vi "Construct Command - Erase.vi"(8 "error in (no error)":errorcluster, 10 "Erase Configuration":T1={"Start Address"="", "End Address"="", "Reset"=TRUE}) -> (0 "error out":errorcluster, 2 "Command":string)   [LabVIEW 2016, in "JLink Commander.lvlib"]
doc: "Construct an Erase command which erases all flash sectors or a certain flash range of the current device. A device has to be specified previously. When specified, all flash between the <SAddr> and <EAddr> will be erased. By default, the device is being reset before starting the erase operation. This may be skipped by adding \"noreset\"."
uses:
  JLink Commander.lvlib
  Type Definitions/Erase Configuration.ctl
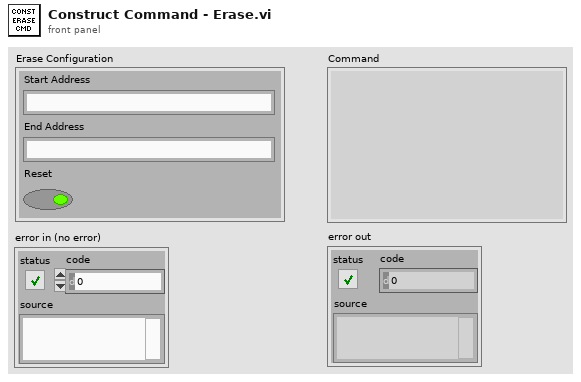
[diagram p1: front panel]
types:
  T1 = typedef "JLink Commander.lvlib/Erase Configuration.ctl" = cluster{"Start Address":string, "End Address":string, "Reset":bool}
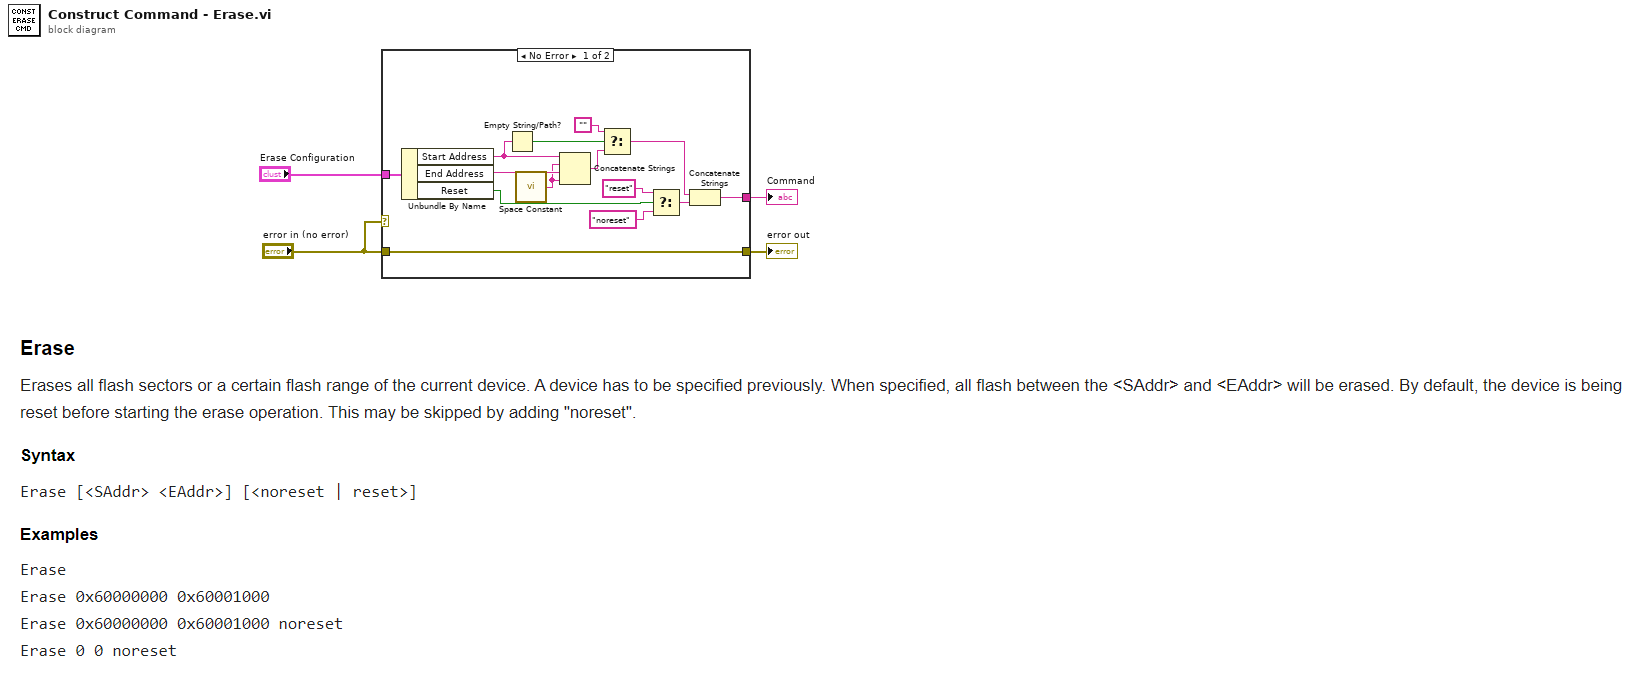
[diagram p0: block diagram]
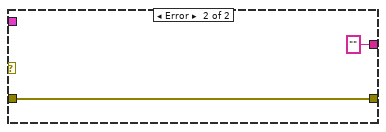
[diagram p2: hidden frame]
diagram:
  n1 = case shown="No Error" "error in (no error)" {
    tunnel: [w17 ""] -> w4
    tunnel: "Erase Configuration" -> [w6 _]
    tunnel: [w5 w19] -> w2
    tunnel: "error in (no error)" -> [w5 w19]
    frame No Error {
      n2 = Unbundle By Name(w6) -> ("Start Address"=w11:string, "End Address"=w12:string, "Reset"=w18:bool)
      n3 = Empty String/Path?(string/path=w11) -> (empty?=w9:bool)
      n4 = call <vilib>:"Space Constant.vi"() -> ("String"=w10:string)
      n5 = Concatenate Strings(w11, w10, w12, w10) -> (w13:string)
      n6 = Select(t="", s=w9, f=w13) -> (s? t:f=w16:string)
      n7 = Select(t="reset", s=w18, f="noreset") -> (s? t:f=w15:string)
      n8 = Concatenate Strings(w16, w15) -> (w17:string)
    }
    frame Error {
    }
  }
  "Command" <- w4
  "error out" <- w2
